vi "Send Graphite Metrics (Polymorphic).vi"   [LabVIEW 2023]
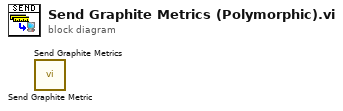
[diagram p0: block diagram]
diagram:
  n1 = call "Send Graphite Metric.vi"() -> ()  [unwired: 8 in, 4 out]
  n2 = call "Send Graphite Metrics.vi"() -> ()  [unwired: 9 in, 3 out]
